vi "CSM - Debug Console2.vi"() -> ()   [LabVIEW 2017]
doc: "CSM Debug Console, you can use this tool:\n\n1. Select an existing CSM instance, open the front panel and block diagram.\n2. Scan the API interfaces of existing CSM instances.\n3. Select an API interface, call synchronously or asynchronously, view the return value.\n4. View the overall program's running log."
uses:
  _Support/Typedef/_CSM_List Module Scope.ctl
  _Support/Typedef/_CSM_GlobalLog_MSG.ctl
  _Support/Typedef/_CSM_Response Source Message.ctl
  _Support/Typedef/_CSM_GlobalLog_MSG_TYPE.ctl
  _jksm/_action.ctl
  1437127e-efa5-494e-aa43-da9d647a7a6f.vi
  6c6a0a0d-4e90-432b-9646-7a8ac0ceadb8.vi
  <vilib>/addons/_JKI Toolkits/State Machine/_JKI_lib_State_Machine.llb/Parse State Queue__JKI_lib_State_Machine.vi
  AdvanceAPI/CSM - Keywords.vi
  AdvanceAPI/CSM - Convert Error to Argument.vi
  _Support/GlobalEvent/GEvt-Generate with Rule Check.vi
  _csmHelper/API/Create From VI Reference.vi
  _csmHelper/API/Update lvcsm Section in VI Description.vi
  _csmHelper/API/Destroy.vi
  _Polymophic/Add State(s) to Queue By BOOL(Element).vi
  _Support/GlobalEvent/Cache-GEvt Refs.vi
  _Support/GlobalEvent/LogFilter/LogFilter - Check.vi
  <vilib>/Utility/Data Type/Get Type Information.vi
  _csmHelper/lvcsmFile/lvcsm File Path.vi
  <vilib>/Utility/config.llb/Open Config Data.vi
  <vilib>/Utility/config.llb/Read Key.vi
  <vilib>/Utility/config.llb/Read Key (Boolean).vi
  <vilib>/Utility/config.llb/Read Key (String).vi
  <vilib>/Utility/Data Type/Get Array Information.vi
  <vilib>/Utility/config.llb/Get Key Names.vi
  _csmHelper/lvcsmFile/Path to lvcsm String.vi
  _csmHelper/lvcsmFile/lvcsm String to Path.vi
  <vilib>/Utility/config.llb/Read Key (I32).vi
  <vilib>/Utility/config.llb/Read Key (Double).vi
  <vilib>/Utility/config.llb/Close Config Data.vi
  _csmHelper/lvcsmFile/_Array of VData to VCluster.vi
  <vilib>/Utility/config.llb/Write Key.vi
  <vilib>/Utility/config.llb/Write Key (Boolean).vi
  <vilib>/Utility/config.llb/Remove Key.vi
  <vilib>/Utility/config.llb/Write Key (String).vi
  <vilib>/Utility/config.llb/Write Key (I32).vi
  <vilib>/Utility/config.llb/Write Key (Double).vi
  _Support/GlobalEvent/LogFilter/LogFilter.lvclass
  Communicable State Machine.lvlib
  _csmHelper/API with lvcsm Support/CSM-Helper API with lvcsm Support.lvlib
  _csmHelper/CSM-Helper.lvclass
  _ui/csm-ui-support.lvlib
  _jksm/_jkism_magic.lvlib
panel:
  in  "Scope":T1
  in  "Refresh CSMs Button":bool
  in  "CSM":string(combo)
  in  "Write lvcsm in Description":bool
  out "inlvlibp":bool
  in  "RetainWireValues":bool
  in  "Toolbar.Exit":bool
  in  "Toolbar.Open FP":bool
  in  "Toolbar.Open BD":bool
  in  "Refresh lvcsm Cache":bool
  in  "History":i32(listbox)
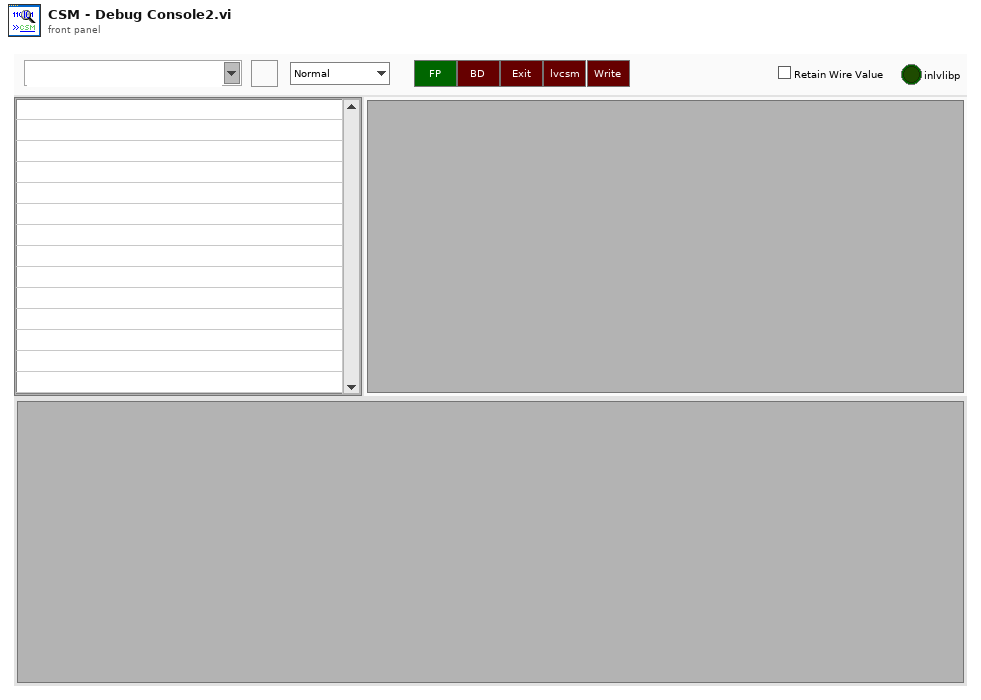
[diagram p1: front panel]
types:
  T1 = typedef "Communicable State Machine.lvlib/_CSM_List Module Scope.ctl" = enum16{"Normal", "System Only", "All"}
  T2 = enum32{"Invalid", "Standard", "Closed", "Hidden", "Minimized", "Maximized"}
  T3 = enum32{"invalid app kind", "Development System", "Run Time System", "Student Edition", "Embedded LabVIEW", "Evaluation", "Custom"}
  T4 = cluster{"Response Timeout(s)":i32, "History Length":i32, "History":string[], "Periodic Enable":bool, "Periodic threashold(#/s)":dbl, "Periodic Check Peroid(s)":dbl}
  T5 = typedef "_jkism_magic.lvlib/_action.ctl" = enum16{"Obtain", "Destroy", "Broadcast", "Post"}
  T6 = cluster{"Shift":bool, "Ctrl":bool, "Alt":bool, "Cmd":bool, "Opt":bool}
  T7 = typedef "LVPoint32TypeDef.ctl" = cluster{"Horizontal":i32, "Vertical":i32}
  T8 = cluster{"Core":cluster{"Current VI Reference":refnum<vi>, "Close Panel on Exit?":bool}, "CSM Global Log Event":refnum<user-event>, "MessageList":string[], "Toobar.advance":refnum<vi>[], "CSM Check History":string[], "History Length":i32}
  T9 = cluster{"Current VI Reference":refnum<vi>, "Close Panel on Exit?":bool}
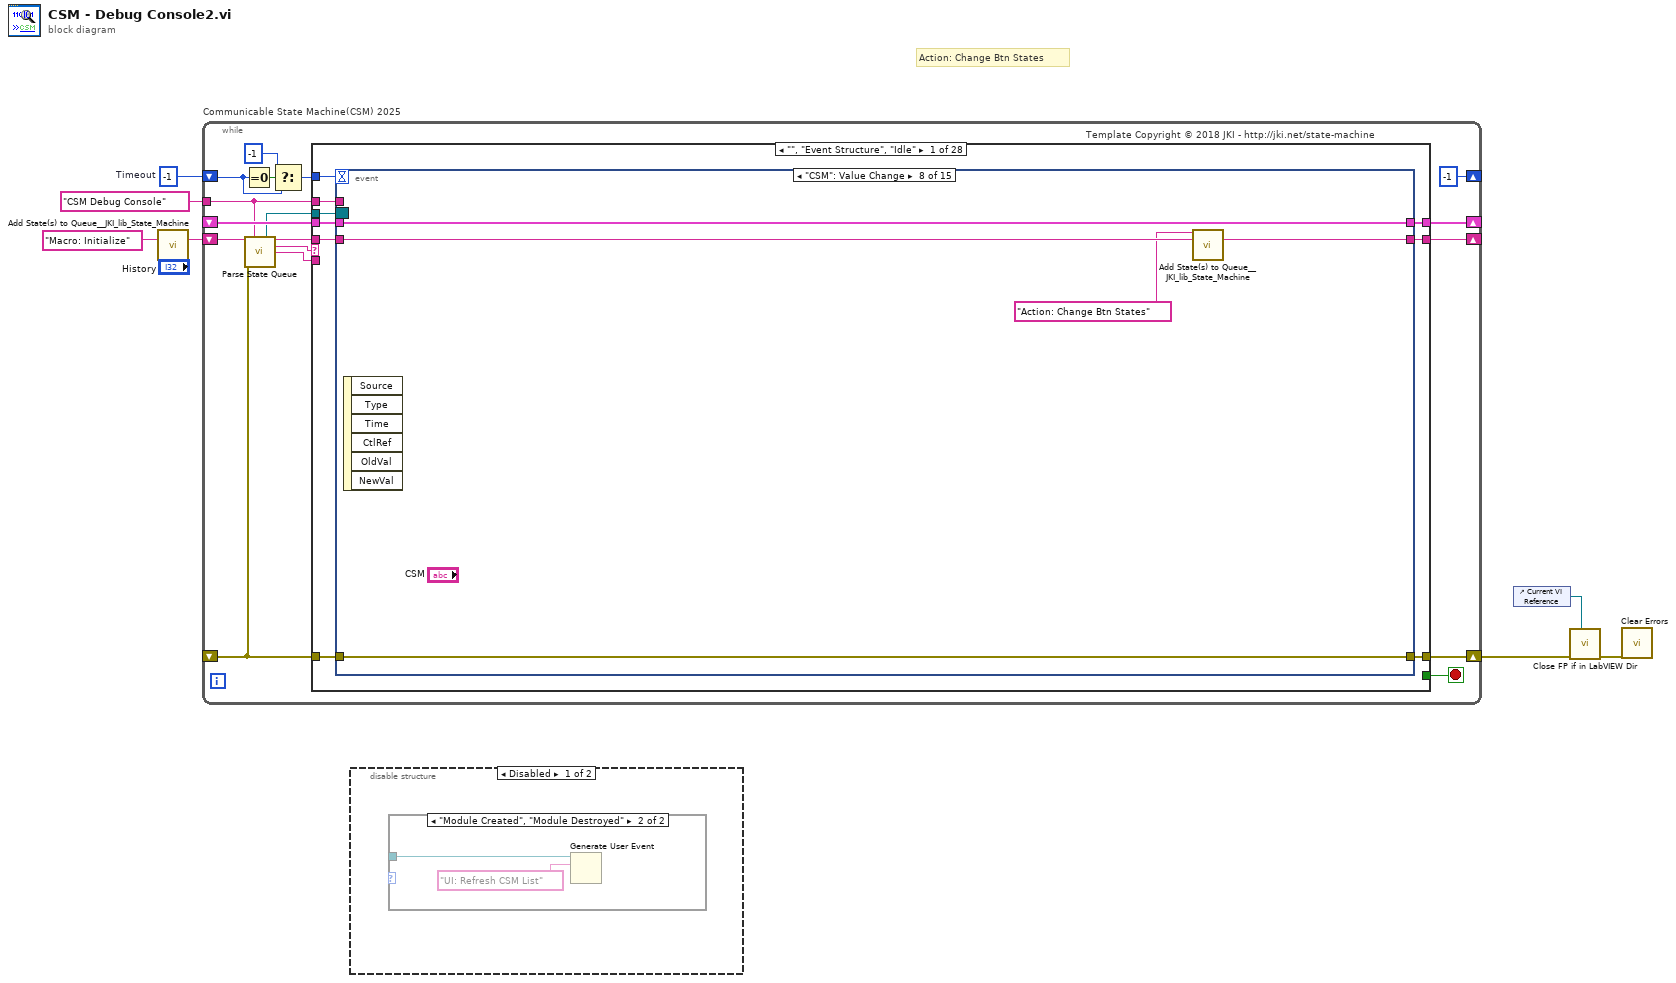
[diagram p0: block diagram]
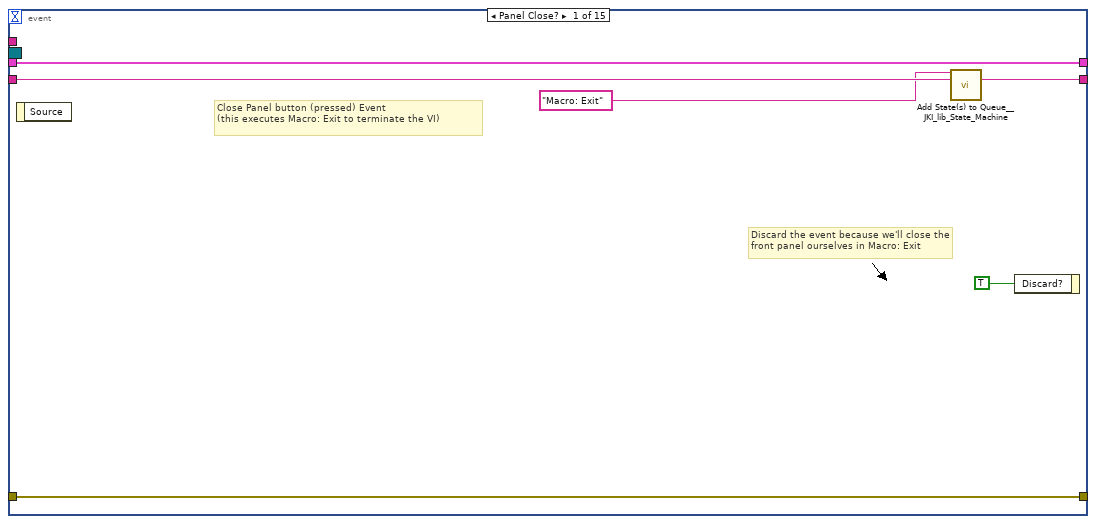
[diagram p4: hidden frame]
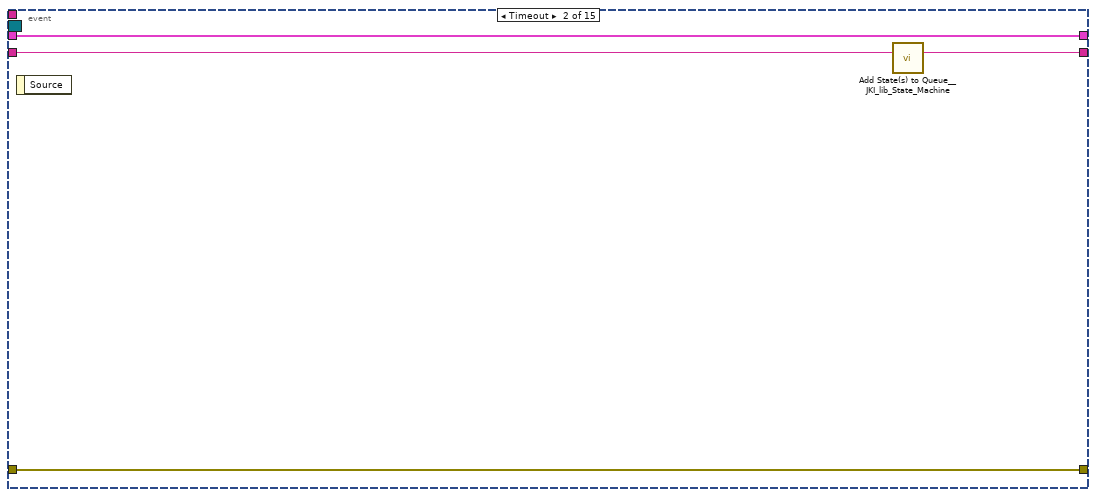
[diagram p5: hidden frame]
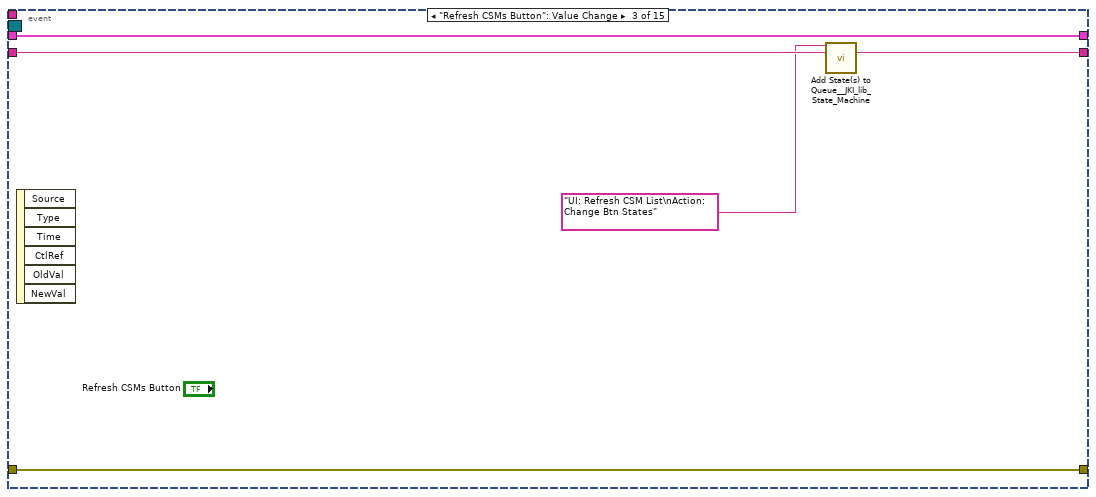
[diagram p6: hidden frame]
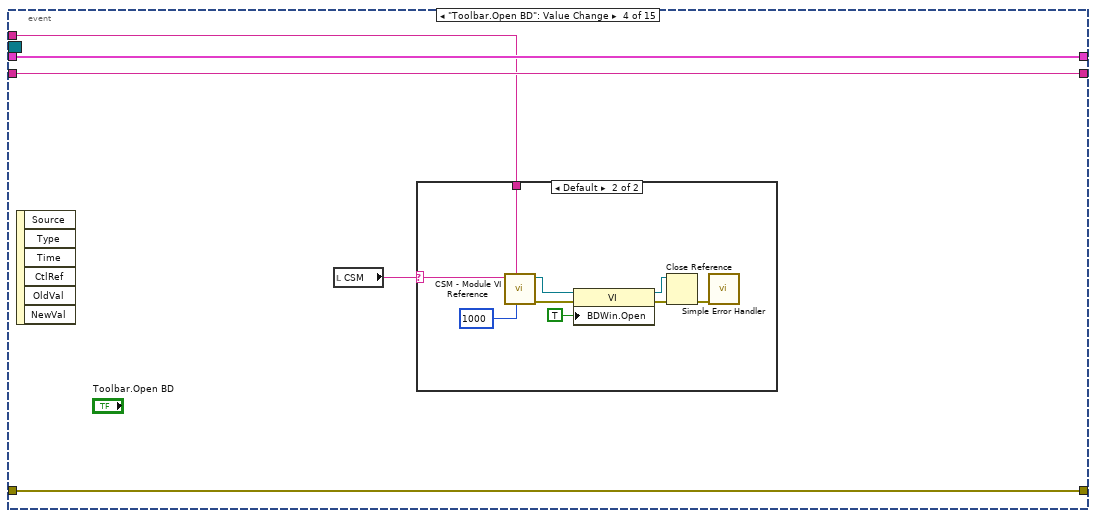
[diagram p7: hidden frame]
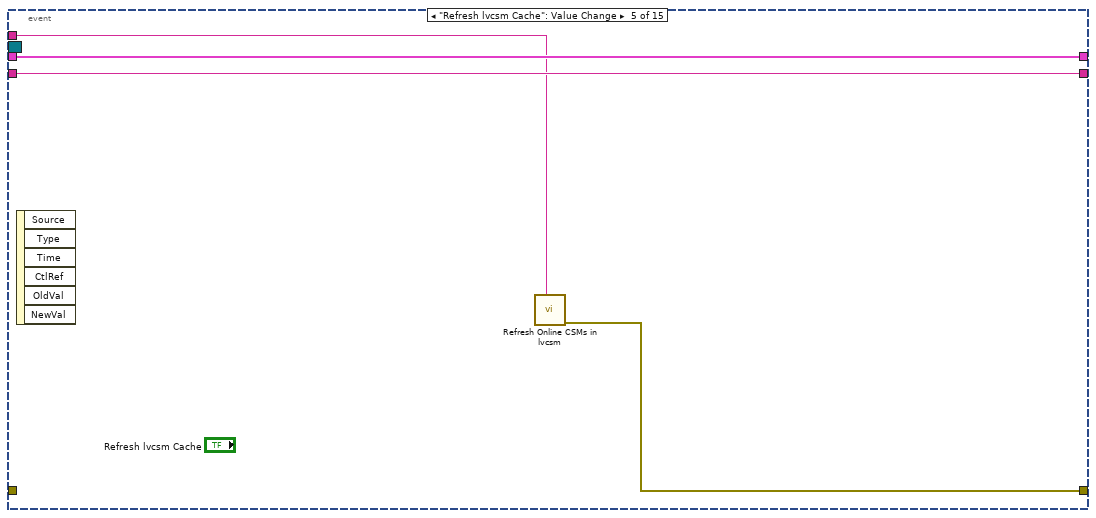
[diagram p9: hidden frame]
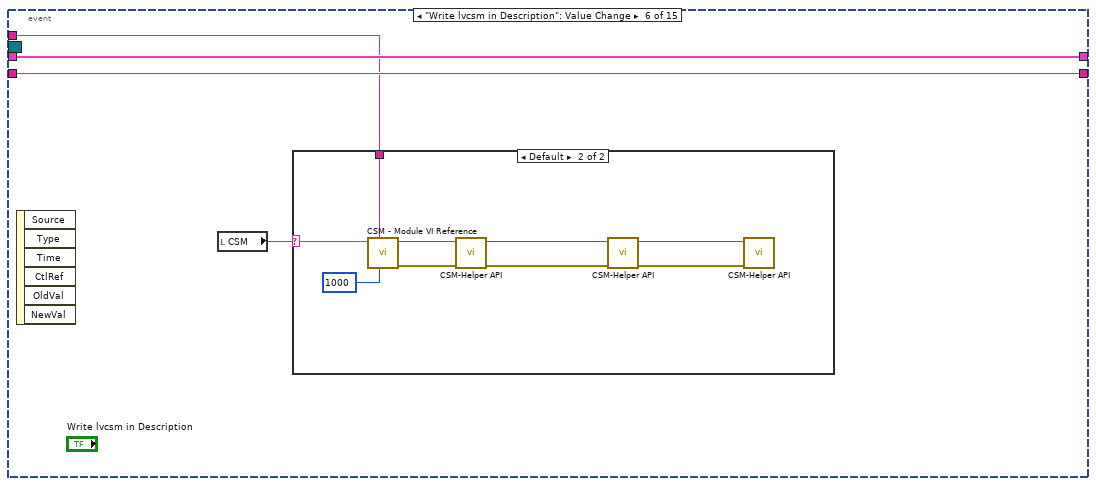
[diagram p10: hidden frame]
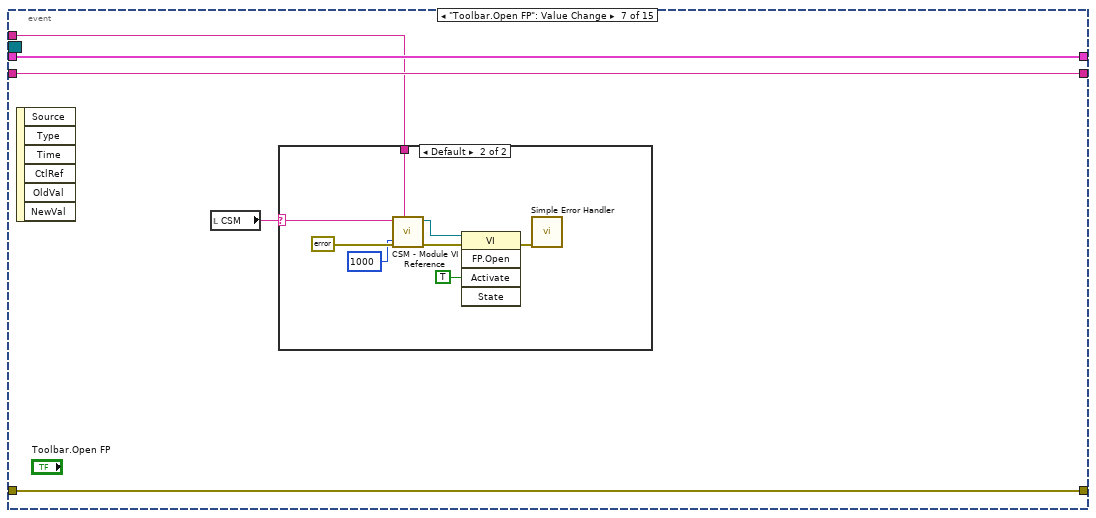
[diagram p12: hidden frame]
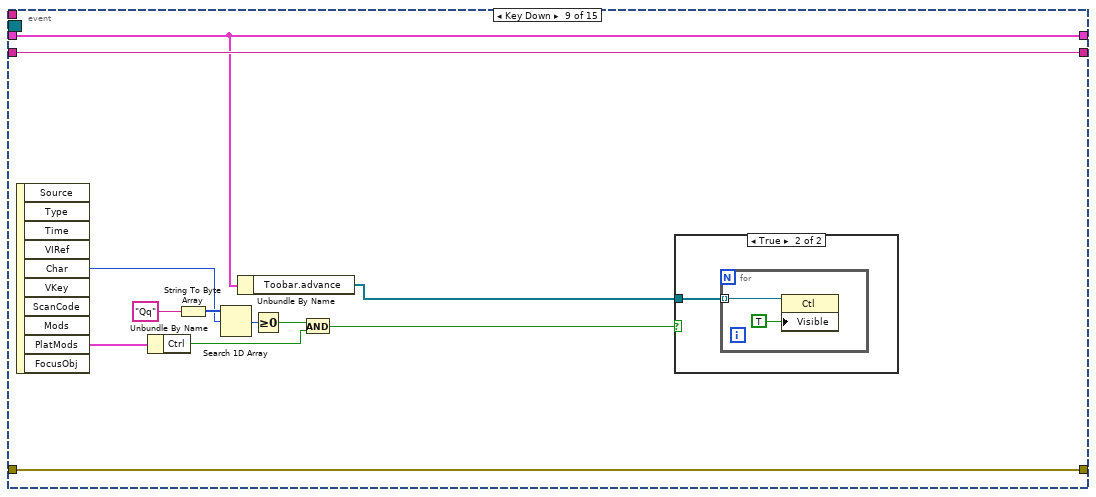
[diagram p14: hidden frame]
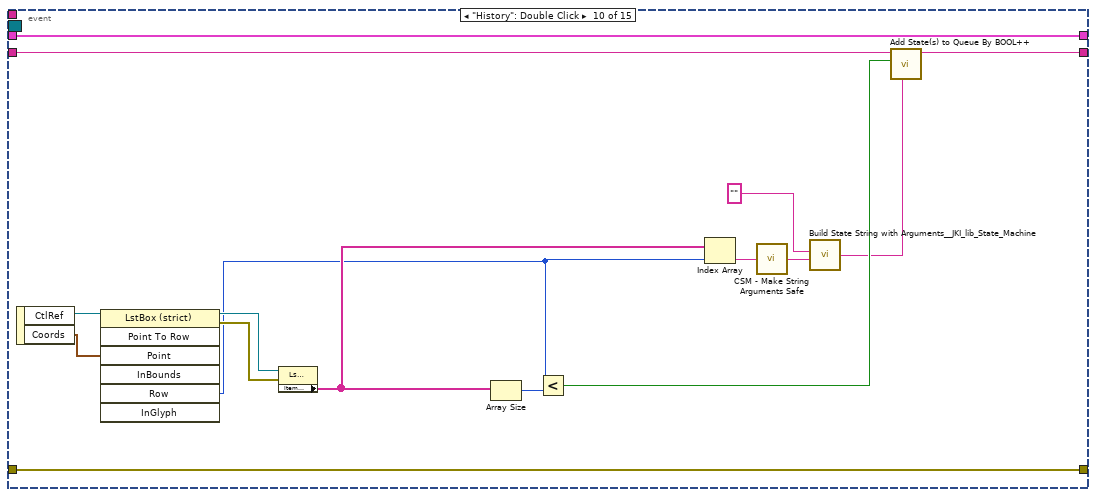
[diagram p16: hidden frame]
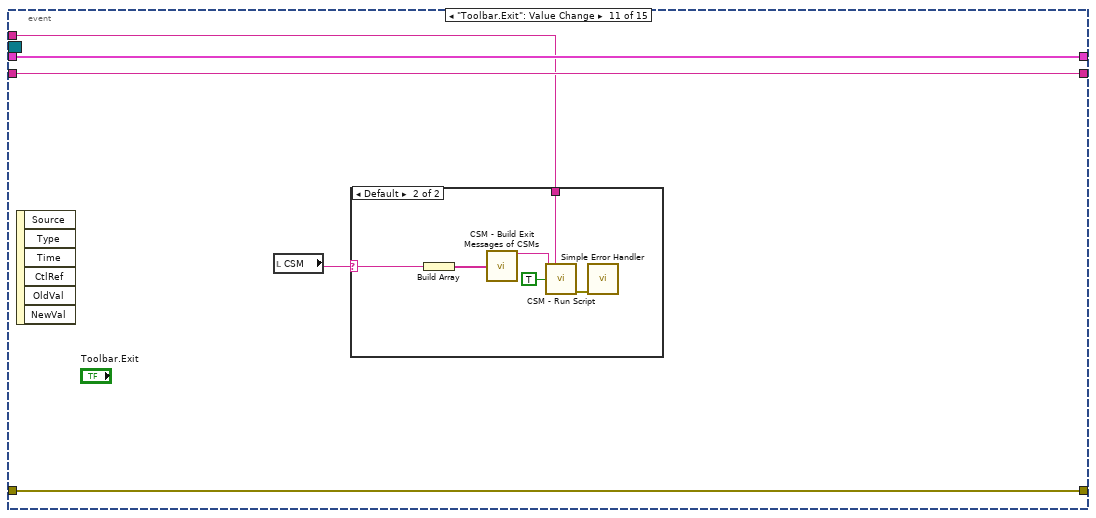
[diagram p17: hidden frame]
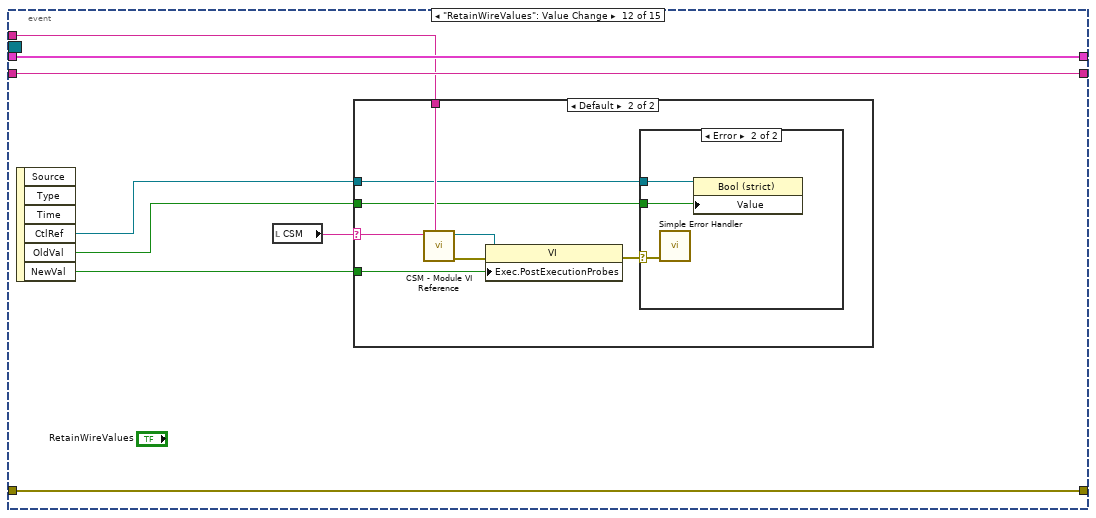
[diagram p19: hidden frame]
diagram:
  w5 = -1  # Timeout
  # "Action: Change Btn States"
  n1 = call <vilib>:"Add State(s) to Queue__JKI_lib_State_Machine.vi"("State(s) in (\"\")"="Macro: Initialize") -> ("States Out"=w6:string)  [unwired: 14 in]
  n2 = while "Communicable State Machine(CSM) 2025" {
    shift-right: [w17] -> _
    shift-left: _ -> [w16]
    shift-right: [w20] -> w2
    shift-left: _ -> [w15]
    shift-right: [w19] -> _
    shift-left: w6 -> [w21]
    tunnel: "CSM Debug Console" -> [w9]
    shift-right: [-1 ("Timeout")] -> _
    shift-left: w5 -> [w12]
    stop <- w18 stop-if-true
    # "Template Copyright © 2018 JKI - http://jki.net/state-machine"
    n3 = Equal To 0?(x=w12) -> (x = 0?=w14:bool)
    n4 = call "Parse State Queue.vi"("State Queue"=w21, "Current Module(\"\" to generate an ID)"=w9, "Error In (no error)"=w15) -> ("Event Registration Refnum"=w8:refnum<event-registration>, "Remaining States"=w23:string, "Current State"=w24:string, "Arguments"=w22:string)  [unwired: 9 in]
    n5 = Select(t=-1 ("Timeout"), s=w14, f=w12) -> (s? t:f=w11:i32)
    n6 = case shown="\"\", \"Event Structure\", \"Idle\"" w24 {
      selector: w24 -> [_ _ w211 _ _ _ _ _ _ _ _ _ _ _ _ _ _ _ _ _ _ _ _ _ _ _ _ _]
      tunnel: w23 -> [w33 w210 w215 w234 w241 w246 w250 w260 w267 w276 w284 w296 w311 w315 w320 w329 w340 w412 w425 w437 w450 w453 w458 w463 w471 w475 w483 w503]
      tunnel: w22 -> [_ _ _ _ _ _ _ _ _ _ _ w292 _ _ _ w324 w334 _ _ _ _ _ _ _ _ _ _ _]
      tunnel: w16 -> [w31 w207 w213 w227 w238 w244 w247 _ w266 w274 w283 w294 w306 w312 w317 w327 w336 w411 w424 w436 w449 w452 w455 w460 w468 w472 w482 w502]
      tunnel: [w30 w208 w217 w231 errorcluster {"status"=FALSE, "code"=0, "source"=""} ("error out") w243 w248 w257 w268 _ w279 w295 w307 w313 w318 w325 w337 w413 w426 w438 w451 w454 w456 w461 w469 w473 w484 w504] -> w20
      tunnel: w15 -> [w29 w208 w216 w231 w237 w243 w248 w257 w268 _ _ w295 w308 w313 w318 w326 w338 w413 w426 w438 w451 w454 w456 w461 w469 w473 w484 w504]
      tunnel: [w32 w209 w214 w233 w240 w245 w249 w259 w267 w276 w284 w296 w310 w314 w319 w328 w339 w412 w425 w437 w450 w453 w457 w462 w470 w474 w483 w503] -> w19
      tunnel: [_ _ _ _ _ TRUE _ _ _ _ _ _ _ _ _ _ _ _ _ _ _ _ _ _ _ _ _ _] -> w18
      tunnel: [w28 w207 w213 w232 w238 w244 w247 w258 w263 w275 w283 w288 w306 w312 w317 w327 w336 w411 w424 w436 w449 w452 w455 w460 w468 w472 w482 w502] -> w17
      tunnel: w11 -> [w27 _ _ _ _ _ _ _ _ _ _ _ _ _ _ _ _ _ _ _ _ _ _ _ _ _ _ _]
      tunnel: w9 -> [w26 _ _ _ w235 _ _ _ _ w272 w280 _ _ _ _ _ _ _ _ _ _ _ _ _ _ _ w480 w500]
      tunnel: w8 -> [w25 _ _ _ _ _ _ _ _ _ _ _ _ _ _ _ _ _ _ _ _ _ _ _ _ _ _ _]
      frame "", "Event Structure", "Idle" {
        n7 = event shown="[7] \"CSM\": Value Change" {
          selector: w25 -> [_ _ _ _ _ _ _ _ _ _ _ _ _ _ _]
          dyn-events: _ -> [_ _ _ _ _ _ _ _ _ _ _ _ _ _ _]
          timeout: w27 -> [_ _ _ _ _ _ _ _ _ _ _ _ _ _ _]
          tunnel: w33 -> [w39 w43 w46 w53 w66 w70 w84 w94 w109 w120 w133 w147 w162 w175 w177]
          tunnel: [w38 w42 w45 w53 w66 w70 w84 w95 w109 w121 w133 w147 w163 w175 w179] -> w32
          tunnel: w31 -> [w36 w40 w47 w52 w65 w69 w83 w96 w98 w127 w132 w145 w164 w173 w180]
          tunnel: [w37 w41 w48 w50 w63 _ w81 w97 w108 w128 w131 w146 w165 w174 w181] -> w30
          tunnel: w29 -> [w37 w41 w48 w50 _ _ w81 w97 w108 w128 w131 w146 w165 w174 w181]
          tunnel: [w36 w40 w47 w52 w65 w69 w83 w96 w98 w127 w132 w145 w164 w173 w178] -> w28
          tunnel: w26 -> [_ _ _ w49 w64 w67 w80 _ _ _ w129 w143 _ _ _]
          event Panel Close? {
            # "Discard the event because we'll close the front panel ourselves in Macro: Exit"
            # "Close Panel button (pressed) Event\n(this executes Macro: Exit to terminate the VI)"
            n8 = event-data() -> ()  [unwired: 1 in, 1 out]
            n9 = call <vilib>:"Add State(s) to Queue__JKI_lib_State_Machine.vi"("State(s) in Front (\"\")"="Macro: Exit", "State(s) in (\"\")"=w39) -> ("States Out"=w38:string)  [unwired: 13 in]
            n10 = event-data("Discard?"=TRUE) -> ()  [unwired: 1 in, 1 out]
          }
          event Timeout {
            n11 = event-data() -> ()  [unwired: 1 in, 1 out]
            n12 = call <vilib>:"Add State(s) to Queue__JKI_lib_State_Machine.vi"("State(s) in (\"\")"=w43) -> ("States Out"=w42:string)  [unwired: 14 in]
          }
          event "Refresh CSMs Button": Value Change {
            n13 = event-data() -> ()  [unwired: 1 in, 6 out]
            n14 = call <vilib>:"Add State(s) to Queue__JKI_lib_State_Machine.vi"("State(s) in Front (\"\")"="UI: Refresh CSM List\nAction: Change Btn States" ("State(s) in Front (\"\")"), "State(s) in (\"\")"=w46) -> ("States Out"=w45:string)  [unwired: 13 in]
          }
          event "Toolbar.Open BD": Value Change {
            n15 = event-data() -> ()  [unwired: 1 in, 6 out]
            n16 = local read "CSM"() -> (w51:string)
            n17 = case shown="Default" w51 {
              selector: w51 -> [_ w61]
              tunnel: w49 -> [_ w60]
              frame "" {
              }
              frame Default {
                n18 = call "CSM - Module VI Reference.vi"("Response Timeout (-2 Using Global Settings)"=1000 ("Response Timeout(5000 ms)"), "Current Module (\"\" to Generate an ID)"=w60, "CSM Name"=w61) -> ("error out"=w54:errorcluster, "CSM Module VIRef"=w59:refnum<vi>)  [unwired: 7 in]
                n19 = property class="VI"(reference=w59, error in=w54, "BDWin.Open"=TRUE ("Block Diagram Window:Open")) -> (reference out=w57:refnum<vi>, error out=w56:errorcluster)
                n20 = Close Reference(reference=w57, error in (no error)=w56) -> (error out=w62:errorcluster)
                n21 = call <vilib>:"Simple Error Handler.vi"("error in (no error)"=w62) -> ()  [unwired: 4 in, 5 out]
              }
            }
          }
          event "Refresh lvcsm Cache": Value Change {
            n22 = event-data() -> ()  [unwired: 1 in, 6 out]
            n23 = call "Refresh Online CSMs in lvcsm.vi"("Caller"=w64) -> ("error out"=w63:errorcluster)  [unwired: 9 in, 1 out]
          }
          event "Write lvcsm in Description": Value Change {
            n24 = event-data() -> ()  [unwired: 1 in, 6 out]
            n25 = local read "CSM"() -> (w68:string)
            n26 = case shown="Default" w68 {
              selector: w68 -> [_ w75]
              tunnel: w67 -> [_ w71]
              frame "" {
              }
              frame Default {
                n27 = call "CSM - Module VI Reference.vi"("Response Timeout (-2 Using Global Settings)"=1000 ("Response Timeout(5000 ms)"), "Current Module (\"\" to Generate an ID)"=w71, "CSM Name"=w75) -> ("error out"=w73:errorcluster, "CSM Module VIRef"=w72:refnum<vi>)  [unwired: 7 in]
                n28 = call-poly "CSM-Helper API.vi"("error in (no error)"=w73, "VI"=w72) -> ("error out"=w79:errorcluster, "CSM-Helper.lvclass"=w78:refnum<class "CSM-Helper.lvclass">)  [unwired: 8 in]
                n29 = call-poly "CSM-Helper API.vi"("error in (no error)"=w79, "CSM-Helper in"=w78) -> ("error out"=w77:errorcluster, "CSM-Helper out"=w76:refnum<class "CSM-Helper.lvclass">)  [unwired: 8 in]
                n30 = call-poly "CSM-Helper API.vi"("error in (no error)"=w77, "CSM-Helper in"=w76) -> ()  [unwired: 8 in, 2 out]
              }
            }
          }
          event "Toolbar.Open FP": Value Change {
            n31 = event-data() -> ()  [unwired: 1 in, 6 out]
            n32 = local read "CSM"() -> (w82:string)
            n33 = case shown="Default" w82 {
              selector: w82 -> [_ w92]
              tunnel: w80 -> [_ w90]
              frame "" {
              }
              frame Default {
                n34 = call "CSM - Module VI Reference.vi"("Response Timeout (-2 Using Global Settings)"=1000 ("Response Timeout(5000 ms)"), "Current Module (\"\" to Generate an ID)"=w90, "error in (no error)"=errorcluster {"status"=FALSE, "code"=0, "source"=""}, "CSM Name"=w92) -> ("error out"=w86:errorcluster, "CSM Module VIRef"=w87:refnum<vi>)  [unwired: 6 in]
                n35 = invoke on="Invoke Node" class="VI" method="FP.Open"(reference=w87, error in=w86, "Activate"=TRUE ("Activate?")) -> (error out=w91:errorcluster)  [unwired: 2 in, 4 out]
                n36 = call <vilib>:"Simple Error Handler.vi"("error in (no error)"=w91) -> ()  [unwired: 4 in, 5 out]
              }
            }
          }
          event "CSM": Value Change {
            n37 = event-data() -> ()  [unwired: 1 in, 6 out]
            n38 = call <vilib>:"Add State(s) to Queue__JKI_lib_State_Machine.vi"("State(s) in Front (\"\")"="Action: Change Btn States" ("State(s) in Front (\"\")"), "State(s) in (\"\")"=w94) -> ("States Out"=w95:string)  [unwired: 13 in]
          }
          event Key Down {
            n39 = event-data() -> ("Char"=w99:i16, "PlatMods"=w100:T6)  [unwired: 1 in, 8 out]
            n40 = Unbundle By Name(w100) -> ("Ctrl"=w103:bool)
            n41 = String To Byte Array(string="Qq") -> (unsigned byte array=w105:u8[])
            n42 = Search 1D Array(1D array=w105, element=w99) -> (index of element=w106:i32)  [unwired: 1 in]
            n43 = Unbundle By Name(w98) -> ("Toobar.advance"=w101:refnum<vi>[])
            n44 = Greater Or Equal To 0?(x=w106) -> (x >= 0?=w107:bool)
            n45 = And(x=w107, y=w103) -> (x .and. y?=w102:bool)
            n46 = case shown="True" w102 {
              tunnel: w101 -> [_ w110]
              frame False {
              }
              frame True {
                n47 = for {
                  tunnel: w110 -> [w112] mode=indexing
                  n48 = property class="Ctl"(reference=w112, "Visible"=TRUE) -> ()  [unwired: 1 in, 2 out]
                }
              }
            }
          }
          event "History": Double Click {
            n49 = event-data() -> ("CtlRef"=w126:refnum<vi>, "Coords"=w114:T7)  [unwired: 1 in]
            n50 = invoke class="LstBox (strict)" method="Point To Row"(reference=w126, "Point"=w114) -> (reference out=w125:refnum<vi>, error out=w124:errorcluster, "Row"=w113:i32)  [unwired: 5 in, 4 out]
            n51 = property class="LstBox (strict)"(reference=w125, error in=w124) -> ("Item Names"=w122:string[])  [unwired: 2 out]
            n52 = Array Size(array=w122) -> (size(s)=w123:i32)
            n53 = Less?(x=w113, y=w123) -> (x < y?=w119:bool)
            n54 = Index Array(array=w122, index=w113) -> (element=w118:string)
            n55 = call "CSM - Make String Arguments Safe.vi"("Argument String"=w118) -> ("Safe Argument String"=w117:string)  [unwired: 8 in]
            n56 = call <vilib>:"Build State String with Arguments__JKI_lib_State_Machine.vi"("Arguments (\"\")"=w117, "State"="") -> ("State with Arguments"=w115:string)  [unwired: 4 in]
            n57 = call-poly "Add State(s) to Queue By BOOL++.vi"("TRUE (\"\")"=w115, "Condition"=w119, "State Queue (\"\")"=w120) -> ("Remaining States"=w121:string)  [unwired: 8 in]
          }
          event "Toolbar.Exit": Value Change {
            n58 = event-data() -> ()  [unwired: 1 in, 6 out]
            n59 = local read "CSM"() -> (w130:string)
            n60 = case shown="Default" w130 {
              selector: w130 -> [_ w136]
              tunnel: w129 -> [_ w139]
              frame "" {
              }
              frame Default {
                n61 = Build Array(w136) -> (w135:string[])
                n62 = call "CSM - Build Exit Messages of CSMs.vi"("CSMs"=w135) -> ("States"=w137:string)  [unwired: 14 in]
                n63 = call "CSM - Run Script.vi"("CSM Scripts"=w137, "Current Module (\"\" to Generate an ID)"=w139, "Continue If Error? (F)"=TRUE) -> ("error out"=w138:errorcluster)  [unwired: 10 in, 2 out]
                n64 = call <vilib>:"Simple Error Handler.vi"("error in (no error)"=w138) -> ()  [unwired: 4 in, 5 out]
              }
            }
          }
          event "RetainWireValues": Value Change {
            n65 = event-data() -> ("CtlRef"=w141:refnum<vi>, "OldVal"=w140:bool, "NewVal"=w142:bool)  [unwired: 1 in, 3 out]
            n66 = local read "CSM"() -> (w144:string)
            n67 = case shown="Default" w144 {
              selector: w144 -> [_ w153]
              tunnel: w143 -> [_ w152]
              tunnel: w142 -> [_ w151]
              tunnel: w141 -> [_ w149]
              tunnel: w140 -> [_ w148]
              frame "" {
              }
              frame Default {
                n68 = call "CSM - Module VI Reference.vi"("Current Module (\"\" to Generate an ID)"=w152, "CSM Name"=w153) -> ("error out"=w155:errorcluster, "CSM Module VIRef"=w154:refnum<vi>)  [unwired: 8 in]
                n69 = property class="VI"(reference=w154, error in=w155, "Exec.PostExecutionProbes"=w151) -> (error out=w150:errorcluster)  [unwired: 1 out]
                n70 = case shown="Error" w150 {
                  selector: w150 -> [_ w156]
                  tunnel: w149 -> [_ w158]
                  tunnel: w148 -> [_ w157]
                  frame No Error {
                  }
                  frame Error {
                    n71 = call <vilib>:"Simple Error Handler.vi"("error in (no error)"=w156) -> ()  [unwired: 4 in, 5 out]
                    n72 = property class="Bool (strict)"(reference=w158, "Value"=w157) -> ()  [unwired: 1 in, 2 out]
                  }
                }
              }
            }
          }
          event User Event {
            n73 = event-data() -> ("JKISM External Event"=w161:string)  [unwired: 1 in, 4 out]
            n74 = call "Pass Allowed Message.vi"("Allowed Message"=string[] ["Macro: Exit", "CSM: Module List Changed"], "JKISM External Event"=w161) -> ("States"=w160:string)  [unwired: 1 in]
            n75 = call <vilib>:"Add State(s) to Queue__JKI_lib_State_Machine.vi"("State(s) in Front (\"\")"=w160, "State(s) in (\"\")"=w162) -> ("States Out"=w163:string)  [unwired: 13 in]
          }
          event "History": Shortcut Menu Activation? {
            n76 = event-data() -> ("MenuRef"=w172:refnum<k9>)  [unwired: 1 in, 6 out]
            n77 = Index Array(array=string[][] [["Set History Length", "SET_HISTORY_LEN_MENU"], ["APP_SEPARATOR", "APP_SEPARATOR"], ["Clear All...", "CLEAR_HISOTRY_MENU"]] ("item names"), index (col) #1=0 ("index (row)"), index (col) #2=1 ("index (row)")) -> (element #1=w170:string[], element #2=w168:string[])  [unwired: 2 in]
            n78 = Insert Menu Items(7:w168, 8:w170, 9:w172) -> ()  [unwired: 3 in, 3 out]
            n79 = event-data("Discard?"=FALSE) -> ()  [unwired: 1 in, 1 out]
          }
          event "History": Shortcut Menu Selection (User) {
            n80 = event-data() -> ("ItemTag"=w176:string)  [unwired: 1 in, 7 out]
            n81 = case shown="\"SET_HISTORY_LEN_MENU\"" w176 {
              tunnel: w180 -> [w183 w190 w199]
              tunnel: [w182 w189 w198] -> w179
              tunnel: [w183 w188 w197] -> w178
              tunnel: w177 -> [w182 w186 w198]
              frame Default {
              }
              frame "CLEAR_HISOTRY_MENU" {
                n82 = Two Button Dialog(message="Clear Command History List?") -> (T button?=w184:bool)  [unwired: 2 in]
                n83 = case shown="True" w184 {
                  tunnel: w190 -> [w191 w194]
                  tunnel: [w191 w193] -> w188
                  frame False {
                  }
                  frame True {
                    n84 = Bundle By Name(cluster=w194, "MessageList"=string[] []) -> (w193:T8)
                  }
                }
                n85 = call-poly "Add State(s) to Queue By BOOL++.vi"("TRUE (\"\")"="UI: Refresh History List" ("State(s) in Front (\"\")"), "Condition"=w184, "State Queue (\"\")"=w186) -> ("Remaining States"=w189:string)  [unwired: 8 in]
              }
              frame "SET_HISTORY_LEN_MENU" {
                n86 = call "Change CSM Debugging History Length"() -> ("History Length"=w196:dbl, "OK"=w195:bool)  [unwired: 17 in, 1 out]
                n87 = case shown="True" w195 {
                  tunnel: w199 -> [w200 w206]
                  tunnel: [w200 w205] -> w197
                  tunnel: w196 -> [_ w203]
                  frame False {
                  }
                  frame True {
                    n88 = To Long Integer(number=w203) -> (32bit integer=w201:i32)
                    n89 = Max & Min(x=w201, y=50) -> (max(x,y)=w204:i32)  [unwired: 1 out]
                    n90 = Bundle By Name(cluster=w206, "History Length"=w204) -> (w205:T8)
                  }
                }
              }
            }
          }
        }
      }
      frame "---------- Core ----------" {
        # "Do not put any code in this frame.\n(it is a separator no-op)"
        n91 = call <vilib>:"Add State(s) to Queue__JKI_lib_State_Machine.vi"("State(s) in (\"\")"=w210) -> ("States Out"=w209:string)  [unwired: 14 in]
      }
      frame Default {
        w220 = 42 items=["No error", "Argument error", "Memory is full", "Out of zone", "End of file", "File already open", "Generic file I/O error", "File not found", "File permission error", "Disk is full", "Duplicate path", "Too many files open", "System feature not enabled", "Resource file not found", "Cannot add resource", "Resource not found", "Image not found", "Image memory error", "Pen does not exist", "Config type invalid", "Config token not found", "Config parse error", "Config memory error", "Bad external code format", "Bad external code offset", "External code not present", "Null window", "Destroy window error", "Null menu", "Print aborted", "Bad print record", "Print driver error", "Windows error during printing", "Memory error during printing", "Print dialog error", "Generic print error", "Invalid device refnum", "Device not found", "Device parameter error", "Device unit error", "Cannot open device", "Device call aborted", "Generic error", "Cancelled by user", "Object ID too low", "Object ID too high", "Object not in heap", "Unknown heap", "Unknown object (invalid DefProc)", "Unknown object (DefProc not in table)", "Message out of range", "Invalid (null) method", "Unknown message", "Manager call not supported", "Bad address", "Network operation in progress", "Network operation timed out", "Connection is busy", "Network attribute not supported", "Network error", "Address in use", "System out of memory", "Connection aborted", "Connection refused", "Not connected", "Already connected", "Connection closed", "Initialization error (interapplication manager)", "Bad occurrence", "Wait on unbound occurrence handler", "Occurrence queue overflow", "Datalog type conflict", "Unused", "Unrecognized type (interapplication manager)", "Memory corrupt", "Failed to make temporary DLL", "Old CIN version", "Drag socket not found", "Failed to load drop-object", "Failed to register OLE object", "Failed to release OLE object", "Format specifier type mismatch", "Unknown format specifier", "Too few format specifiers", "Too many format specifiers", "Scan failed", "Newer CIN version", "Error converting to variant", "Runtime menu error", "Password tampered", "Variant attribute not found", "Incompatible variant data type", "Event data is not available", "Event Store is not present", "Occurrence is not found", "Event Queue is not created", "Event info is not available", "Refnum passed is NULL", "Error retrieving Class GUID", "Error retrieving CoClass GUID", "Error retrieving TypeLib GUID.", "Bad built application magic bytes.", "Specific driver is different from the specific driver associated with the Logical Name.", "There is no session opened to the class driver.", "Max Error", "MAX - Error with config objects", "MAX - Error loading configuration", "MAX - Group not supported"]
        # "Current State"
        # "Do not delete, rename, or modify this frame.\n(this is used to capture unhandled states and typos)"
        # "Handle mistyped state name (developer tool)"
        n92 = Format Into String(format string="Software Exception: Unhandled State \"%s\"." ("message"), error in=w216, w211) -> (resulting string=w219:string, error out=w218:errorcluster)  [unwired: 1 in]
        n93 = call <vilib>:"Error Cluster From Error Code.vi"("show call chain? (False)"=TRUE, "error in (no error)"=w218, "error message (\"\")"=w219, "error code (0)"=w220) -> ("error out"=w217:errorcluster)  [unwired: 5 in]
        n94 = call <vilib>:"Add State(s) to Queue__JKI_lib_State_Machine.vi"("State(s) in (\"\")"=w215) -> ("States Out"=w214:string)  [unwired: 14 in]
      }
      frame "Initialize Core Data" {
        # "Do not delete, rename, or modify this frame.\n(this is used to determine panel behavior on exit)"
        # "originally closed?"
        # "exe?"
        # "If panel starts closed or is an EXE, then close it when we exit"
        n95 = property class="VI"() -> ("FP.State"=w224:T2)  [unwired: 2 in, 2 out]
        n96 = property class="App"() -> ("App.Kind"=w230:T3)  [unwired: 2 in, 2 out]
        n97 = control-ref of="Current VI Reference"() -> (w225:refnum<vi>)
        n98 = Equal?(x=w224, y=T2."Closed" ("Front Panel Window:State")) -> (x = y?=w222:bool)
        n99 = Equal?(x=w230, y=T3."Run Time System" ("Application:Kind")) -> (x = y?=w228:bool)
        n100 = Or(x=w222, y=w228) -> (x .or. y?=w226:bool)
        n101 = Bundle By Name(cluster=w227, "Core.Current VI Reference"=w225, "Core.Close Panel on Exit?"=w226) -> (w232:T8)
        n102 = call <vilib>:"Add State(s) to Queue__JKI_lib_State_Machine.vi"("State(s) in (\"\")"=w234) -> ("States Out"=w233:string)  [unwired: 14 in]
      }
      frame "Error Handler" {
        # "Unhandled Error -- Display it"
        # "Handle any errors here.\nYou can also output any states to clean-up after errors occur"
        # "Clear error"
        n103 = call "CSM - Global Log Error Handler.vi"("Place (\"\" to Use VI's Name)"=w235, "Error In"=w237) -> ()  [unwired: 9 in, 1 out]
        n104 = call <vilib>:"Add State(s) to Queue__JKI_lib_State_Machine.vi"("State(s) in Front (\"\")"="/* Post Error States", "State(s) in (\"\")"=w241) -> ("States Out"=w240:string)  [unwired: 13 in]
      }
      frame "Exit" {
        # "Do not put any code in this frame.\n(No errors that occur here will be handled.)"
        n105 = call <vilib>:"Add State(s) to Queue__JKI_lib_State_Machine.vi"("State(s) in (\"\")"=w246) -> ("States Out"=w245:string)  [unwired: 14 in]
      }
      frame "---------- Data ----------" {
        # "Do not put any code in this frame.\n(It is a separator no-op. You can make a copy of this frame to create a new Data frame)"
        n106 = call <vilib>:"Add State(s) to Queue__JKI_lib_State_Machine.vi"("State(s) in (\"\")"=w250) -> ("States Out"=w249:string)  [unwired: 14 in]
      }
      frame "Data: Initialize" {
        w251 = 50  # History Length
        w252 = string[] []  # CSM Check History
        w253 = refnum<vi>[] []  # Toobar.advance
        w254 = string[] []  # MessageList
        w255 = refnum<user-event> refnum  # CSM Global Log Event
        w256 = T9 {"Current VI Reference"=refnum, "Close Panel on Exit?"=FALSE}  # Core
        # "Initialize the shift-register data, here.\n(data names are defined by what you wire into the bundle function)"
        n107 = Bundle("Core"=w256, "CSM Global Log Event"=w255, "MessageList"=w254, "Toobar.advance"=w253, "CSM Check History"=w252, "History Length"=w251) -> (w258:T8)  [unwired: 1 in]
        n108 = call <vilib>:"Add State(s) to Queue__JKI_lib_State_Machine.vi"("State(s) in (\"\")"=w260) -> ("States Out"=w259:string)  [unwired: 14 in]
      }
      frame "Data: Initialize References" {
        n109 = control-ref of="Toolbar.Open FP"() -> (w265:refnum<vi>)
        n110 = control-ref of="Toolbar.Open BD"() -> (w264:refnum<vi>)
        n111 = control-ref of="Refresh lvcsm Cache"() -> (w261:refnum<vi>)
        n112 = Build Array(w265, w264, w261) -> (w262:refnum<vi>[])
        n113 = Bundle By Name(cluster=w266, "Toobar.advance"=w262) -> (w263:T8)
      }
      frame "Data: Load Arguments Config File" {
        n114 = call "lvcsm Read Cluster.vim"("Section"=w272, "Default Prototype"=T4 {"Response Timeout(s)"=30, "History Length"=50, "History"=[], "Periodic Enable"=TRUE, "Periodic threashold(#/s)"=0.5, "Periodic Check Peroid(s)"=3.0}) -> ("Cluster (Dup)"=w273:T4)  [unwired: 8 in, 1 out]
        n115 = Unbundle By Name(w273) -> ("History Length"=w269:i32, "History"=w271:string[])  [unwired: 4 out]
        n116 = Bundle By Name(cluster=w274, "History Length"=w269, "MessageList"=w271) -> (w275:T8)
      }
      frame "Data: Save Arguments Config File" {
        n117 = Unbundle By Name(w283) -> ("MessageList"=w281:string[], "History Length"=w277:i32)
        n118 = Bundle By Name(cluster=T4 {"Response Timeout(s)"=30, "History Length"=50, "History"=[], "Periodic Enable"=TRUE, "Periodic threashold(#/s)"=0.5, "Periodic Check Peroid(s)"=3.0}, "History"=w281, "History Length"=w277) -> (w282:T4)
        n119 = call "lvcsm Write Cluster.vim"("Section"=w280, "Configuration"=w282) -> ("error out"=w279:errorcluster)  [unwired: 9 in]
      }
      frame "Data: Update Message List" {
        n120 = Unbundle By Name(w294) -> ("MessageList"=w293:string[], "History Length"=w285:i32)
        n121 = call "CSM - Revert Arguments-Safe String.vi"("Safe Argument String"=w292) -> ("Origin Argument String"=w291:string)  [unwired: 8 in]
        n122 = Build Array (concatenate)(w291, w293) -> (w290:string[])
        n123 = for {
          tunnel: w290 -> [w300] mode=indexing
          shift-right: [w299] -> w286
          shift-left: string[] [] -> [w298]
          i -> [w297]
          n124 = Search 1D Array(1D array=w298, element=w300) -> (index of element=w301:i32)  [unwired: 1 in]
          n125 = case shown="-1" w301 {
            tunnel: w300 -> [_ w305]
            tunnel: [w302 w303] -> w299
            tunnel: w298 -> [w302 w304]
            tunnel: w297 -> [_ _]
            frame Default {
            }
            frame -1 {
              n126 = Build Array (concatenate)(w304, w305) -> (w303:string[])
            }
          }
        }
        n127 = Array Subset(array=w286, length=w285) -> (w287:string[])  [unwired: 1 in]
        n128 = Bundle By Name(cluster=w294, "MessageList"=w287) -> (w288:T8)
      }
      frame "Data: Cleanup" {
        # "Cleanup any data and references, here.\n(this is called automatically, by the Macro: Exit)"
        n129 = Unbundle By Name(w306) -> ("Core.Current VI Reference"=w309:refnum<vi>)
        n130 = Close Reference(reference=w309, error in (no error)=w308) -> (error out=w307:errorcluster)
        n131 = call <vilib>:"Add State(s) to Queue__JKI_lib_State_Machine.vi"("State(s) in (\"\")"=w311) -> ("States Out"=w310:string)  [unwired: 14 in]
      }
      frame "---------- UI ----------" {
        # "Do not put any code in this frame.\n(It is a separator no-op. You can make a copy of this frame to create a new UI frame)"
        n132 = call <vilib>:"Add State(s) to Queue__JKI_lib_State_Machine.vi"("State(s) in (\"\")"=w315) -> ("States Out"=w314:string)  [unwired: 14 in]
      }
      frame "UI: Initialize" {
        # "Initialize the User Interface, here.\n(this is called automatically, by the Macro: Init)"
        n133 = Unbundle By Name(w317) -> ("Toobar.advance"=w316:refnum<vi>[])
        n134 = disable-structure shown="Disabled" {
          disable-tunnel: w316 -> [w321 _]
          frame Disabled {
            n135 = for {
              tunnel: w321 -> [w323] mode=indexing
              n136 = property class="Ctl"(reference=w323, "Visible"=FALSE) -> ()  [unwired: 1 in, 2 out]
            }
          }
          frame Enabled {
          }
        }
        n137 = call <vilib>:"Add State(s) to Queue__JKI_lib_State_Machine.vi"("State(s) in (\"\")"=w320) -> ("States Out"=w319:string)  [unwired: 14 in]
      }
      frame "UI: Cursor Set" {
        # "Argument"
        # "Set and Unset Cursor Busy.\n(Usage: \"UI: Cursor Set >> Busy|Idle\")"
        n138 = case shown="\"Idle\", Default" w324 {
          tunnel: w326 -> [w331 w333]
          tunnel: [w330 w332] -> w325
          frame "Idle", Default {
            n139 = call <vilib>:"Unset Busy.vi"("error in (no error)"=w331) -> ("error out"=w330:errorcluster)  [unwired: 10 in]
          }
          frame "Busy" {
            n140 = call <vilib>:"Set Busy.vi"("error in (no error)"=w333) -> ("error out"=w332:errorcluster)  [unwired: 9 in, 1 out]
          }
        }
        n141 = call <vilib>:"Add State(s) to Queue__JKI_lib_State_Machine.vi"("State(s) in (\"\")"=w329) -> ("States Out"=w328:string)  [unwired: 14 in]
      }
      frame "UI: Front Panel State" {
        # "Argument"
        # "Set Front Panel Open or Closed\n(Usage: \"UI: Front Panel State >> Open|Close\")"
        n142 = Unbundle By Name(w336) -> ("Core.Current VI Reference"=w335:refnum<vi>)
        n143 = case shown="\"Minimize\", \"Minimized\"" w334 {
          tunnel: w338 -> [w346 w361 w372 w385 w398]
          tunnel: [w348 w362 w374 w387 w400] -> w337
          tunnel: w335 -> [w347 w359 w373 w386 w399]
          frame "Open", "Standard", Default {
            w341 = T2."Standard" ("State")
            n144 = property class="VI"(reference=w347, error in=w346) -> (reference out=w344:refnum<vi>, error out=w345:errorcluster, "FP.State"=w343:T2)
            n145 = Not Equal?(x=w343, y=w341) -> (x != y?=w342:bool)
            n146 = case shown="True" w342 {
              tunnel: [w352 w354] -> w348
              tunnel: w345 -> [w351 w354]
              tunnel: w344 -> [w350 _]
              tunnel: w341 -> [w349 _]
              frame True {
                n147 = invoke class="VI" method="FP.Open"(reference=w350, error in=w351, "Activate"=TRUE, "State"=w349) -> (error out=w352:errorcluster)  [unwired: 1 in, 4 out]
              }
              frame False {
              }
            }
          }
          frame "Close", "Closed" {
            n148 = property class="VI"(reference=w359, error in=w361) -> (reference out=w358:refnum<vi>, error out=w360:errorcluster, "FP.State"=w356:T2)
            n149 = Not Equal?(x=w356, y=T2."Closed" ("Front Panel Window:State")) -> (x != y?=w355:bool)
            n150 = case shown="True" w355 {
              tunnel: [w363 w366] -> w362
              tunnel: w360 -> [w363 w365]
              tunnel: w358 -> [_ w364]
              frame False {
              }
              frame True {
                n151 = invoke class="VI" method="FP.Close"(reference=w364, error in=w365) -> (error out=w366:errorcluster)  [unwired: 1 in, 2 out]
              }
            }
          }
          frame "Hidden", "Hide" {
            w367 = T2."Hidden" ("State")
            n152 = property class="VI"(reference=w373, error in=w372) -> (reference out=w370:refnum<vi>, error out=w371:errorcluster, "FP.State"=w369:T2)
            n153 = Not Equal?(x=w369, y=w367) -> (x != y?=w368:bool)
            n154 = case shown="True" w368 {
              tunnel: [w378 w379] -> w374
              tunnel: w371 -> [w377 w379]
              tunnel: w370 -> [w376 _]
              tunnel: w367 -> [w375 _]
              frame True {
                n155 = invoke class="VI" method="FP.Open"(reference=w376, error in=w377, "State"=w375) -> (error out=w378:errorcluster)  [unwired: 2 in, 4 out]
              }
              frame False {
              }
            }
          }
          frame "Minimize", "Minimized" {
            w380 = T2."Minimized" ("State")
            n156 = property class="VI"(reference=w386, error in=w385) -> (reference out=w383:refnum<vi>, error out=w384:errorcluster, "FP.State"=w382:T2)
            n157 = Not Equal?(x=w382, y=w380) -> (x != y?=w381:bool)
            n158 = case shown="True" w381 {
              tunnel: [w391 w392] -> w387
              tunnel: w384 -> [w390 w392]
              tunnel: w383 -> [w389 _]
              tunnel: w380 -> [w388 _]
              frame True {
                n159 = invoke class="VI" method="FP.Open"(reference=w389, error in=w390, "State"=w388) -> (error out=w391:errorcluster)  [unwired: 2 in, 4 out]
              }
              frame False {
              }
            }
          }
          frame "Maximize", "Maximized" {
            w393 = T2."Maximized" ("State")
            n160 = property class="VI"(reference=w399, error in=w398) -> (reference out=w396:refnum<vi>, error out=w397:errorcluster, "FP.State"=w395:T2)
            n161 = Not Equal?(x=w395, y=w393) -> (x != y?=w394:bool)
            n162 = case shown="True" w394 {
              tunnel: [w404 w405] -> w400
              tunnel: w397 -> [w403 w405]
              tunnel: w396 -> [w402 _]
              tunnel: w393 -> [w401 _]
              frame True {
                n163 = invoke class="VI" method="FP.Open"(reference=w402, error in=w403, "State"=w401) -> (error out=w404:errorcluster)  [unwired: 2 in, 4 out]
              }
              frame False {
              }
            }
          }
        }
        n164 = call <vilib>:"Add State(s) to Queue__JKI_lib_State_Machine.vi"("State(s) in (\"\")"=w340) -> ("States Out"=w339:string)  [unwired: 14 in]
      }
      frame "UI: Refresh History List" {
        n165 = Unbundle By Name(w411) -> ("MessageList"=w408:string[])
        n166 = property on="History" class="LstBox (strict)"() -> ("Item Names"=w409:string[], "Value"=w410:i32)  [unwired: 2 in, 2 out]
        n167 = Index Array(array=w409, index=w410) -> (element=w406:string)
        n168 = Search 1D Array(1D array=w408, element=w406) -> (index of element=w407:i32)  [unwired: 1 in]
        n169 = property on="History" class="LstBox (strict)"("Item Names"=w408, "Value"=w407) -> ()  [unwired: 2 in, 2 out]
      }
      frame "CSM: Module List Changed", "UI: Refresh CSM List" {
        n170 = control-ref of="CSM"() -> (w423:refnum<vi>)
        n171 = property on="Property Node" class="CmbBox"(reference=w423) -> (reference out=w415:refnum<vi>, "Value"=w419:string)  [unwired: 1 in, 1 out]
        n172 = call "CSM - List Modules.vi"("Scope (Normal)"="Scope") -> ("error out"=w422:errorcluster, "Module Names"=w417:string[])  [unwired: 9 in]
        n173 = Search 1D Array(1D array=w417, element=w419) -> (index of element=w421:i32)  [unwired: 1 in]
        n174 = Greater Or Equal To 0?(x=w421) -> (x >= 0?=w420:bool)
        n175 = Index Array(array=w417) -> (element=w418:string)  [unwired: 1 in]
        n176 = Select(t=w419, s=w420, f=w418) -> (s? t:f=w416:string)
        n177 = call <vilib>:"Simple Error Handler.vi"("error in (no error)"=w422) -> ()  [unwired: 4 in, 5 out]
        n178 = property on="Property Node" class="CmbBox"(reference=w415, "Strings[]"=w417, "Val(Sgnl)"=w416) -> ()  [unwired: 1 in, 2 out]
      }
      frame "UI: Insert LogViewer" {
        # "Replace with your own CSM Module"
        n179 = vi-ref "CSM - LogViewer2.vi"() -> (w429:refnum<vi>)
        n180 = property class="VI Interface Type 1"(reference=w429) -> (reference out=w433:refnum<vi>, error out=w431:errorcluster, "Path"=w430:path)  [unwired: 1 in]
        n181 = Open VI Reference(type specifier VI Refnum (for type only)=w433, vi path=w430, options=128, error in (no error)=w431) -> (vi reference=w432:refnum<vi>, error out=w428:errorcluster)  [unwired: 2 in]
        n182 = call-by-ref "Start Asynchronous Call"(reference=w432, error in=w428) -> (reference out=w427:refnum<vi>, error out=w434:errorcluster)  [unwired: 12 in]
        n183 = Close Reference(reference=w427, error in (no error)=w434) -> ()  [unwired: 1 out]
        n184 = invoke on="subpnl" class="SubPnl" method="Insert VI"("VI Ref"=w427) -> ()  [unwired: 3 in, 4 out]
      }
      frame "UI: Insert Message Console" {
        # "Replace with your own CSM Module"
        n185 = vi-ref "CSM - Message Console.vi"() -> (w442:refnum<vi>)
        n186 = property class="VI Interface Type 1"(reference=w442) -> (reference out=w446:refnum<vi>, error out=w444:errorcluster, "Path"=w443:path)  [unwired: 1 in]
        n187 = Open VI Reference(type specifier VI Refnum (for type only)=w446, vi path=w443, options=128, error in (no error)=w444) -> (vi reference=w445:refnum<vi>, error out=w441:errorcluster)  [unwired: 2 in]
        n188 = call-by-ref "Start Asynchronous Call"(reference=w445, error in=w441) -> (reference out=w440:refnum<vi>, error out=w447:errorcluster)  [unwired: 12 in]
        n189 = Close Reference(reference=w440, error in (no error)=w447) -> ()  [unwired: 1 out]
        n190 = control-ref of="subpnl"() -> (w439:refnum<vi>)
        n191 = invoke on="Invoke Node" class="SubPnl" method="Insert VI"(reference=w439, "VI Ref"=w440) -> ()  [unwired: 2 in, 4 out]
      }
      frame "UI: Refresh UI" {
      }
      frame "---------- Macro ----------" {
        # "Do not put any code in this frame.\n(It is a separator no-op. You can make a copy of this frame to create a new Macro frame)"
        n192 = call <vilib>:"Add State(s) to Queue__JKI_lib_State_Machine.vi"("State(s) in (\"\")"=w458) -> ("States Out"=w457:string)  [unwired: 14 in]
      }
      frame "Macro: Initialize" {
        # "Initialization Macro\n(This is called once, when the VI starts)"
        n193 = call <vilib>:"Add State(s) to Queue__JKI_lib_State_Machine.vi"("State(s) in Front (\"\")"="Data: Initialize\nData: Initialize References\nInitialize Core Data\nUI: Initialize\nData: Load Arguments Config File\nUI: Front Panel State >> Open\nUI: Insert Message Console\nUI: Insert LogViewer\nUI: Refresh CSM List\nUI: Refresh History List\nUI: Refresh UI\nAction: Change Btn States", "State(s) in (\"\")"=w463) -> ("States Out"=w462:string)  [unwired: 13 in]
      }
      frame "Macro: Exit" {
        # "Exit Macro\n(This is called once, when the VI exits)"
        n194 = call "FGV-JKISM Modules.vi"("Enum"=_action."Broadcast", "Message"="Macro: Exit") -> ()  [unwired: 8 in, 2 out]
        n195 = call <vilib>:"Add State(s) to Queue__JKI_lib_State_Machine.vi"("State(s) at Back (\"\")"="Data: Save Arguments Config File\nData: Cleanup\nExit") -> ("States Out"=w466:string)  [unwired: 14 in]
        n196 = call <vilib>:"Add State(s) to Queue__JKI_lib_State_Machine.vi"("State(s) in Front (\"\")"=w466, "State(s) in (\"\")"=w471) -> ("States Out"=w470:string)  [unwired: 13 in]
      }
      frame "---------- Action ----------" {
        # "Template Separator\n(You can make a copy of, or modify, this frame)"
        n197 = call <vilib>:"Add State(s) to Queue__JKI_lib_State_Machine.vi"("State(s) in (\"\")"=w475) -> ("States Out"=w474:string)  [unwired: 14 in]
      }
      frame "Action: Change Btn States" {
        n198 = local read "CSM"() -> (w481:string)
        n199 = local read "CSM"() -> (w478:string)
        n200 = call <vilib>:"Build State String with Arguments__JKI_lib_State_Machine.vi"("Arguments (\"\")"=w478, "State"="CSM: Module Selected" ("Message")) -> ("State with Arguments"=w479:string)  [unwired: 4 in]
        n201 = call "FGV-JKISM Modules.vi"("Enum"=_action."Broadcast", "Message"=w479) -> ()  [unwired: 8 in, 2 out]
        n202 = case shown="Default" w481 {
          selector: w481 -> [_ w499]
          tunnel: w480 -> [_ w498]
          frame "" {
          }
          frame Default {
            n203 = call "CSM - Module VI Reference.vi"("Response Timeout (-2 Using Global Settings)"=1000 ("Response Timeout(5000 ms)"), "Current Module (\"\" to Generate an ID)"=w498, "error in (no error)"=errorcluster {"status"=FALSE, "code"=0, "source"=""}, "CSM Name"=w499) -> ("error out"=w494:errorcluster, "CSM Module VIRef"=w495:refnum<vi>)  [unwired: 6 in]
            n204 = property class="VI"(reference=w495, error in=w494) -> (reference out=w488:refnum<vi>, "IsInPackedLibrary"=→"inlvlibp":bool, "Diagram"=w487:refnum<vi>)  [unwired: 1 out]
            n205 = Not A Number/Path/Refnum?(number/path/refnum=w487) -> (NaN/Path/Refnum?=w491:bool)
            n206 = Select(t=2, s=w491, f=0) -> (s? t:f=w492:i32)
            n207 = Close Reference(reference=w487) -> (error out=w486:errorcluster)  [unwired: 1 in]
            n208 = call <vilib>:"Clear Errors.vi"("error in (no error)"=w486) -> ("error out"=w485:errorcluster)  [unwired: 5 in, 1 out]
            n209 = property on="Toolbar.Open BD" class="Bool"("DisabledEnum"=w492) -> ()  [unwired: 2 in, 2 out]
            n210 = Close Reference(reference=w488, error in (no error)=w485) -> ()  [unwired: 1 out]
          }
        }
      }
      frame "No Peroidic Log over 1s" {
        n211 = call "CSM - Generate User Global Log.vi"("Place (\"\" to Use VI's Name)"=w500, "Log"="No Peroidic Log over 1s.") -> ()  [unwired: 9 in, 1 out]
      }
    }
  }
  n212 = disable-structure shown="Disabled" {
    frame Disabled {
      n213 = case shown="\"Module Created\", \"Module Destroyed\"" {
        selector: _ -> [_ _]
        tunnel: _ -> [_ w506]
        frame "User Log", Default {
        }
        frame "Module Created", "Module Destroyed" {
          n214 = Generate User Event(user event=w506, event data cluster="UI: Refresh CSM List" ("State(s) in Front (\"\")")) -> ()  [unwired: 2 in, 2 out]
        }
      }
    }
    frame Enabled {
    }
  }
  n215 = control-ref of="Current VI Reference"() -> (w3:refnum<vi>)
  n216 = call "Close FP if in LabVIEW Dir.vi"("VI Refnum"=w3, "Error in"=w2) -> ("Error out"=w4:errorcluster)  [unwired: 9 in]
  n217 = call <vilib>:"Clear Errors.vi"("error in (no error)"=w4) -> ()  [unwired: 5 in, 2 out]
